vi "Decimal-Converter.vi"() -> ()   [LabVIEW 2014]
panel:
  out "binary":string
  in  "stop":bool
  out "Hexadecimal":string
  out "Octal":string
  in  "Decimal input":i32
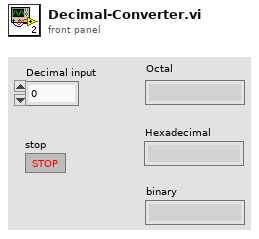
[diagram p1: front panel]
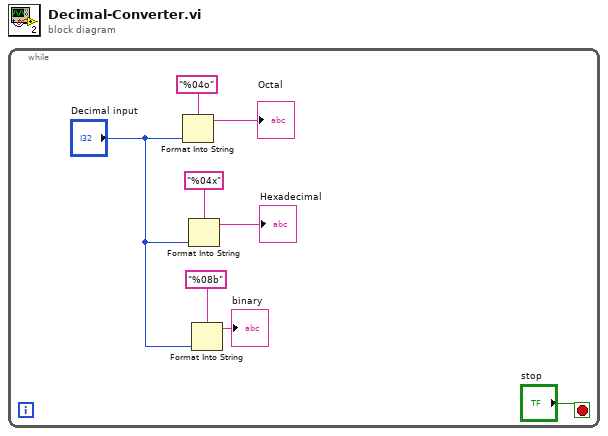
[diagram p0: block diagram]
diagram:
  n1 = while {
    stop <- "stop" stop-if-true
    n2 = Format Into String(format string="%04o", "Decimal input") -> (resulting string=→"Octal":string)  [unwired: 2 in, 1 out]
    n3 = Format Into String(format string="%04x", "Decimal input") -> (resulting string=→"Hexadecimal":string)  [unwired: 2 in, 1 out]
    n4 = Format Into String(format string="%08b", "Decimal input") -> (resulting string=→"binary":string)  [unwired: 2 in, 1 out]
  }
